vi "mono2rgb_hologram.vi"(4 "Force?":bool, 6 "pySession":refnum<k35>, 7 "monoHolo":T1=refnum, 8 "True hologram?":bool=TRUE, 9 "SLM brand":string(combo)="SanTec", 10 "Holo2slm in":T1=refnum, 11 "Holo2show in":T1=refnum) -> (2 "Holo2slm out":T1, 3 "Holo2show out":T1)   [LabVIEW 2023]
uses:
  <vilib>/vision/Image Controls.llb/IMAQ Image.ctl
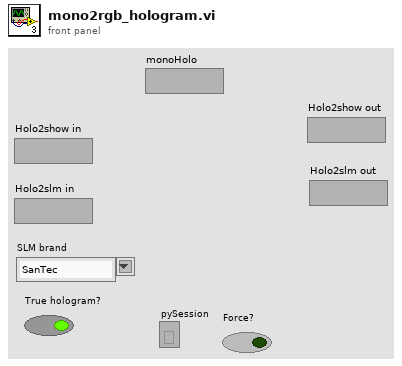
[diagram p1: front panel]
types:
  T1 = typedef "IMAQ Image.ctl" = refnum<image>
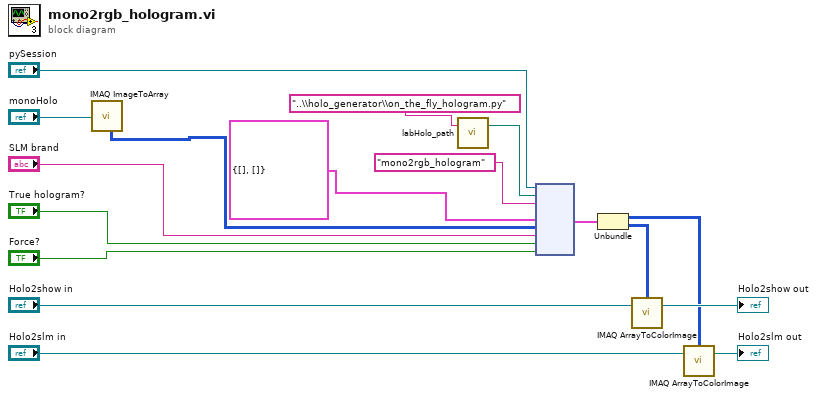
[diagram p0: block diagram]
diagram:
  n1 = call "IMAQ ImageToArray"("Image"="monoHolo") -> ("Image Pixels (U16)"=w1:u16[][])  [unwired: 3 in, 4 out]
  n2 = call "labHolo_path.vi"("sub folder or file (str)"="..\\holo_generator\\on_the_fly_hologram.py") -> ("labHolo path"=w14:path)  [unwired: 1 in, 1 out]
  n3 = node("pySession", w14, "mono2rgb_hologram" ("function name"), cluster{u32[][], u32[][]} {[], []}, w1, "SLM brand", "True hologram?", "Force?") -> (w6:cluster{u32[][], u32[][]})  [unwired: 5 in, 4 out]
  n4 = Unbundle(w6) -> (w2:u32[][], w3:u32[][])
  n5 = call "IMAQ ArrayToColorImage"("Image Pixels (U32)"=w3, "Image"="Holo2show in") -> ("Image Out"=→"Holo2show out":T1)  [unwired: 3 in, 1 out]
  n6 = call "IMAQ ArrayToColorImage"("Image Pixels (U32)"=w2, "Image"="Holo2slm in") -> ("Image Out"=→"Holo2slm out":T1)  [unwired: 3 in, 1 out]
